vi "Read Config File.vi"(8 "error in (no error)":errorcluster, 10 "Car Option":string[](array[string]), 11 "Database in":refnum<class "Database.lvclass">) -> (0 "error out":errorcluster, 3 "Database out":refnum<class "Database.lvclass">)   [LabVIEW 2015, in "Database.lvlib" / "Database.lvclass"]
uses:
  Database.lvclass
  <vilib>/ActorFramework/Actor/Actor.lvclass/Actor.ctl
  Database.lvclass/Database.ctl
  Controls/Wash Option Parameter.ctl
  Controller/Controller Messages/Get Wash Parameters Msg/Get Wash Parameters Msg.lvclass/Get Wash Parameters Msg.ctl
  <vilib>/ActorFramework/Message Enqueuer/Message Enqueuer.lvclass/Message Enqueuer.ctl
  <vilib>/ActorFramework/Message Enqueuer/Enqueue.vi
  <vilib>/Utility/config.llb/Read Key (I32).vi
  <vilib>/Utility/config.llb/Read Key (Double).vi
  <vilib>/ActorFramework/Message Priority Queue/Priority Enqueue.vi
  Controller/Controller Messages/Get Wash Parameters Msg/Get Wash Parameters Msg.lvclass
  <vilib>/Utility/config.llb/NI_LVConfig.lvlib
  <vilib>/ActorFramework/Actor/Actor.lvclass
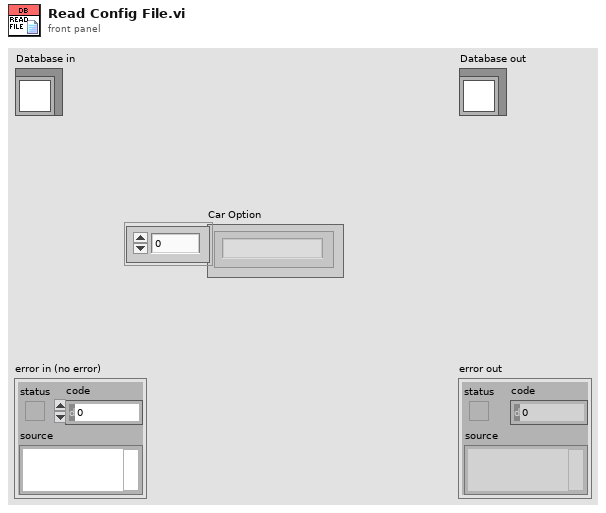
[diagram p1: front panel]
types:
  T1 = typedef "Wash Option Parameter.ctl" = cluster{"Station Name":string, "Station":i32, "Delay":dbl}
  T2 = typedef "NI_LVConfig.lvlib/Config Data RefNum.ctl" = refnum<k1>
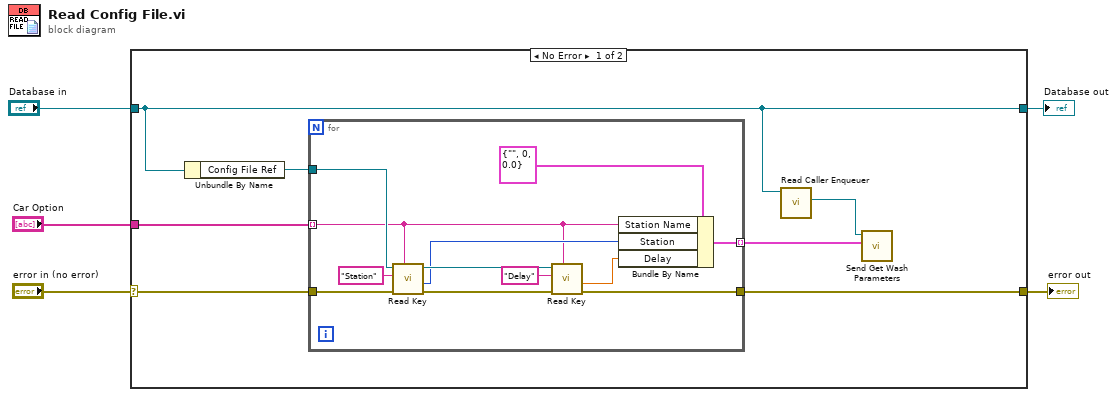
[diagram p0: block diagram]
diagram:
  n1 = case shown="No Error" "error in (no error)" {
    selector: "error in (no error)" -> [w11 w26]
    tunnel: [w10 w26] -> w4
    tunnel: [w8 w25] -> w2
    tunnel: "Database in" -> [w8 w25]
    tunnel: "Car Option" -> [w12 _]
    frame No Error {
      n2 = Unbundle By Name(w8) -> ("Config File Ref"=w9:T2)
      n3 = for {
        tunnel: w12 -> [w15] mode=indexing
        tunnel: w11 -> [w24]
        tunnel: [w22] -> w10
        tunnel: w9 -> [w21]
        tunnel: [w13] -> w6 mode=indexing
        n4 = call-poly <vilib>:"Read Key.vi"("section"=w15, "error in (no error)"=w24, "key"="Station", "refnum"=w21) -> ("error out"=w23:errorcluster, "value"=w16:i32, "refnum out"=w20:T2)  [unwired: 4 in, 1 out]
        n5 = call-poly <vilib>:"Read Key.vi"("section"=w15, "error in (no error)"=w23, "key"="Delay", "refnum"=w20) -> ("error out"=w22:errorcluster, "value"=w14:dbl)  [unwired: 4 in, 2 out]
        n6 = Bundle By Name(cluster=T1 {"Station Name"="", "Station"=0, "Delay"=0.0} ("Option Parameter"), "Station Name"=w15, "Station"=w16, "Delay"=w14) -> (w13:T1)
      }
      n7 = call <vilib>:"Read Caller Enqueuer.vi"("Actor"=w8) -> ("Caller Enqueuer"=w7:refnum<class "Message Enqueuer.lvclass">)  [unwired: 10 in]
      n8 = call "Send Get Wash Parameters.vi"("Wash Parameters"=w6, "Message Enqueuer"=w7) -> ()  [unwired: 8 in, 2 out]
    }
    frame Error {
    }
  }
  "error out" <- w4
  "Database out" <- w2
